vi "ASI Get Start Pos.vi"(9 "piStartY":i32, 10 "piStartX":i32, 11 "iCameraID":i32) -> (1 "piStartY out":i32, 2 "piStartX out":i32, 3 "function return":i32)   [LabVIEW 2023, in "ASICamera2_no_err.lvlib"]
doc: "ASICAMERA_API ASI_ERROR_CODE ASIGetStartPos(int iCameraID, int *piStartX, int *piStartY);"
uses:
  ASICamera2_no_err.lvlib
  ASICamera2.dll
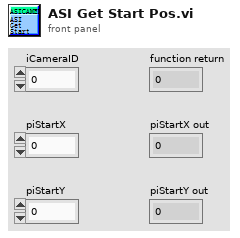
[diagram p1: front panel]
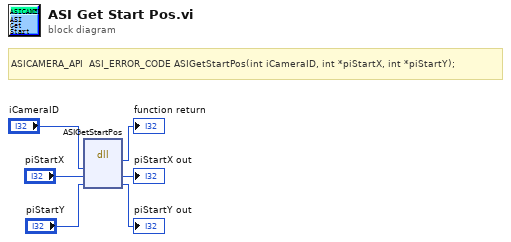
[diagram p0: block diagram]
diagram:
  # "ASICAMERA_API  ASI_ERROR_CODE ASIGetStartPos(int iCameraID, int *piStartX, int *piStartY);"
  n1 = dll-call lib="C:/Users/quantum/Documents/LVDAQ/ConcreteClasses/ConcreteInstrumentClasses/CameraClasses/ZWO_ASI_LV/Labview_ASI_demo_64bit_221128/user.lib/ASICamera2_no_err/ASICamera2.*" fn="ASIGetStartPos"("iCameraID"="iCameraID", "piStartX"="piStartX", "piStartY"="piStartY") -> (→"function return":i32, "piStartX"=→"piStartX out":i32, "piStartY"=→"piStartY out":i32)  [unwired: 4 in, 2 out]
